vi "writeRPDO.vi"(7 "RPDO data":u8[](array[numeric])=[0, 0, 0, 0, 0, 0, 0, 0], 8 "error in (no error)":errorcluster, 9 "PDOChannel":u8(ring) items=["PDO 1", "PDO 2", "PDO 3", "PDO 4"], 10 "interface object in":refnum<k20>, 11 "MotorController in":refnum<class "MotorController.lvclass">) -> (0 "error out":errorcluster, 2 "interface object out":refnum<k20>, 3 "MotorController out":refnum<class "MotorController.lvclass">)   [LabVIEW 2017, in "MotorController.lvclass"]
uses:
  MotorController.lvclass
  MotorController.lvclass/MotorController.ctl
  <vilib>/CANopenLib/CANOPEN.llb/CANopen RPDO Create.vi
  <vilib>/CANopenLib/CANOPEN.llb/CANopen RPDO Start.vi
  <vilib>/CANopenLib/CANOPEN.llb/CANopen RPDO Close.vi
  <resource>/objmgr/CANopenPDO.rc
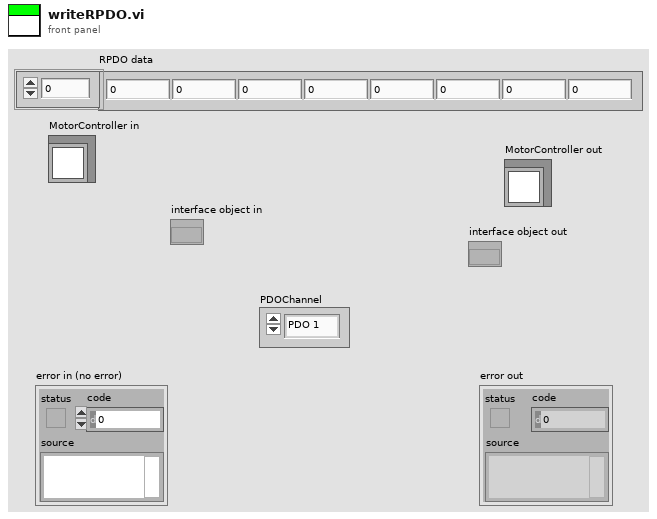
[diagram p1: front panel]
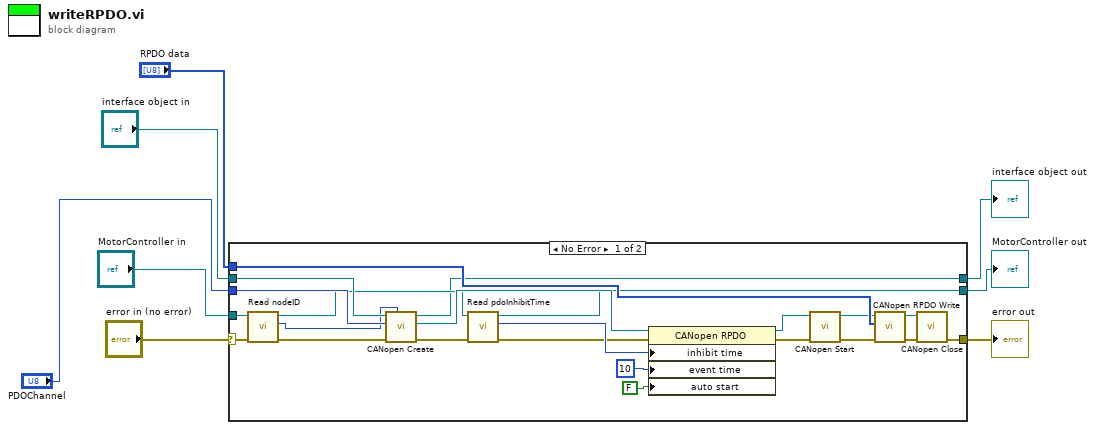
[diagram p0: block diagram]
diagram:
  n1 = case shown="No Error" "error in (no error)" {
    selector: "error in (no error)" -> [w28 w34]
    tunnel: [w13 w34] -> w7
    tunnel: [w9 w33] -> w5
    tunnel: "MotorController in" -> [w29 w33]
    tunnel: [w10 w32] -> w4
    tunnel: "interface object in" -> [w31 w32]
    tunnel: "PDOChannel" -> [w30 _]
    tunnel: "RPDO data" -> [w15 _]
    frame No Error {
      n2 = call "Read nodeID.vi"("error in (no error)"=w28, "MotorController in"=w29) -> ("error out"=w27:errorcluster, "nodeID"=w26:u8, "MotorController out"=w24:refnum<class "MotorController.lvclass">)  [unwired: 7 in]
      n3 = call-poly <vilib>:"CANopen Create.vi"("node-ID"=w26, "error in (no error)"=w27, "PDO channel"=w30, "interface object in"=w31) -> ("error out"=w23:errorcluster, "RPDO object out"=w25:refnum<k20>, "interface object out"=w10:refnum<k20>)  [unwired: 5 in]
      n4 = call "Read pdoInhibitTime.vi"("error in (no error)"=w23, "MotorController in"=w24) -> ("error out"=w19:errorcluster, "pdoInhibitTime"=w22:u8, "MotorController out"=w9:refnum<class "MotorController.lvclass">)  [unwired: 7 in]
      n5 = property class="CANopen RPDO"(reference=w25, error in=w19, "inhibit time"=w22, "event time"=u8 10, "auto start"=FALSE) -> (reference out=w17:refnum<k20>, error out=w18:errorcluster)
      n6 = call-poly <vilib>:"CANopen Start.vi"("error in (no error)"=w18, "RPDO object in"=w17) -> ("error out"=w16:errorcluster, "RPDO object out"=w14:refnum<k20>)  [unwired: 8 in]
      n7 = call <vilib>:"CANopen RPDO Write.vi"("error in (no error)"=w16, "data"=w15, "RPDO object in"=w14) -> ("error out"=w12:errorcluster, "RPDO object out"=w11:refnum<k20>)  [unwired: 7 in]
      n8 = call-poly <vilib>:"CANopen Close.vi"("error in (no error)"=w12, "RPDO object in"=w11) -> ("error out"=w13:errorcluster)  [unwired: 9 in]
    }
    frame Error {
    }
  }
  "error out" <- w7
  "MotorController out" <- w5
  "interface object out" <- w4
